vi "DFD FXP Code Generator.vi"   [LabVIEW 2017, in "NI_DigFilterLicensed.lvlib"]
doc: "Generates fixed-point code from a fixed-point filter, including fixed-point LabVIEW field-programmable gate array (FPGA) code, integer LabVIEW code, and C code. You must manually select the polymorphic instance you want to use."
uses:
  <vilib>/addons/Digital Filter Design/NI_DigFilterLicensed.lvlib
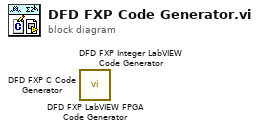
[diagram p0: block diagram]
diagram:
  n1 = call <vilib>:"DFD FXP LabVIEW FPGA Code Generator.vi"() -> ()  [unwired: 9 in, 3 out]
  n2 = call <vilib>:"DFD FXP Integer LabVIEW Code Generator.vi"() -> ()  [unwired: 10 in, 2 out]
  n3 = call <vilib>:"DFD FXP C Code Generator.vi"() -> ()  [unwired: 10 in, 2 out]
